vi "pure pursuit.vi"(8 "input cluster":T3={"Drive Forward Input "=0.0, "Drive Twist Input"=0.0, "Drive Output"=0.0, "Drivetwist Output"=0.0, "Left Joystick Buttons"=[FALSE, FALSE, FALSE, FALSE, FALSE, FALSE, FALSE, FALSE, FALSE, FALSE, FALSE, FALSE], "Left Joystick Axis"=[-0.007874015748031496, -0.007874015748031496, -0.0, -1.0], "Right Joystick Axis"=[], "Right Joystick Button"=[], "Arm Encoder"=102.0, "Left Drive Encoder"=2433.0, "Right Drive Encoder"=6910.0, "Gyro Angle "=3.1201171875, "Arm Joystick Output  "=0.0, "Line Follower L, C, R "=[TRUE, TRUE, TRUE], "Line follow?"=FALSE, " Climb Solenoid"=FALSE, "Wrist Encoder Count"=0.0, "Wrist Joystick Output"=0.0, "Ball Encoder Count"=0.0, "Ball Output"=0.0, "Climb Encoder"=0.0, "Climb Motor Output"=0.0, " Hatch Solenoid"=FALSE, "Arm Setpoint "=6.0, "Wrist Setpoint "=0.0, "Arm Joystick Enabled?"=FALSE, "Wrist Joystick Enabled"=FALSE, "Vision String"="", "Left Joystick POVs"=[-1]}, 10 "Vision Data":dbl[](array[numeric]), 11 "Button":bool) -> ()   [LabVIEW 2018]
uses:
  TypeDefs/Teleop Data Cluster.ctl
  path data.ctl
  TypeDefs/typedef_enum_Refnums.ctl
  <vilib>/Rock Robotics/WPI/Utilities/WPI_GetSetVariantRefNum.vi
  <vilib>/Rock Robotics/Network Tables/NT Write Number.vi
  <vilib>/Rock Robotics/WPI/RobotDrive/WPI_RobotDriveArcadeDrive_Standard(NoSaturation).vi
  <vilib>/Rock Robotics/WPI/ThirdParty/Phoenix-LabVIEW/Pigeon IMU/CTRE_PigeonIMU_GetYPR.vi
  <vilib>/ptbypt/NI_PtbyPt.lvlib
panel:
  in  "Extension Weight":dbl=40.0
  in  "Vision Data 2":dbl[](array[numeric])=[100.0, 30.0, 30.0]
  in  "Reverse?":bool
  in  "End Weight":dbl=40.0
  in  "Start Weight":dbl=40.0
  in  "Path Data":T1={"Path"=[], "Target Velocities"=[], "Robot Location"=[0.0, 0.0], "Relative Robot Angle (rad)"=0.0, "Curvature"=0.0, "Lookahead Point"=[0.0, 0.0], "Lookahead Index"=0.0, "Closest Point"=[0.0, 0.0], "Closest Point Index"=0, "Left Velocity"=0.0, "Right Velocity"=0.0, "Left Encoder Vel"=0, "Right Encoder Vel"=0, "Left Encoder Pos"=0, "Right Encoder Pos"=0, "Inital Robot Angle (deg)"=0.0}
  out "error out":errorcluster
  in  "error in":errorcluster
  in  "Diagnostic?":bool=TRUE
  in  "Tuning":T2={"Kv Left"=0.00023, "Kv Right"=0.00023, "Kp Left"=0.0002, "Kp Right"=0.0002}
  out "Loop Time":u32=49
  out "Exp. Curvature":dbl[](graph)=[0.0, 2.1457073059547978e-06, 4.915984271433975e-06, 9.188824286615022e-06, 1.6525472937545946e-05, 3.010957284935173e-05, 5.6788339571684504e-05, 8.289028577213488e-05, 4.477325703165674e-05, 2.456450460867463e-05, 1.378521585638589e-05, 7.731043410757915e-06, 4.074850806979229e-06, 1.5874818402303252e-06, 4.987974022052938e-07, 2.8449815610461093e-06, 6.3492936805341935e-06, 1.2856441230110154e-05, 2.7535758537289207e-05, 3.0160147141967202e-05, 1.4511775279263373e-05, 7.708104280674182e-06, 4.314732936015046e-06, 2.452638698362967e-06, 1.3278260165247803e-06, 5.18742643953799e-07, 0.0]
  out "Curvature":dbl(graph)=-0.0001411444266515344
  out "Target Velocities":cluster{dbl, dbl}(graph)
  in  "Lookahead Distance":dbl=5000.0 format="%#_13g"
  out "Path":T4(graph)=[{"Smooth Path"=[0.0, 183.6988592949273, 380.76323574317996, 607.8995296360172, 889.3325158488149, 1262.8611917273658, 1789.308518427094, 2567.7266854376426, 3771.076875333013, 5232.402820741672, 6849.244028409719, 8558.017396302117, 10318.123190930659, 12101.795305964908, 13887.15873864522, 15652.761438127307, 17372.21087078327, 19007.57686157632, 20499.90780396381, 21754.493387203354, 23022.702335030026, 24295.5868812136, 25565.368128084057, 26823.491402011234, 28058.487557976674, 29253.105583025565, 30379.999999999993], "Smooth Path"=[0.0, 2562.5448292081915, 5114.539619045078, 7642.796141488607, 10128.191737636604, 12540.888817075378, 14832.875496937382, 16925.961760858292, 18910.53913716453, 20828.576963041232, 22705.412156107523, 24556.078957478312, 26389.070280301727, 28208.460788155666, 30014.92415836178, 31805.902606457305, 33574.96665674355, 35310.20911679595, 36991.26656448049, 38584.22946121987, 40426.874048932084, 42415.21298923889, 44481.68243571063, 46578.25117050202, 48664.41284268002, 50697.05928458697, 52619.7035339425]}, {"Smooth Path"=[24052.273982374318, 27574.516343499825], "Smooth Path"=[40888.03333583952, 45745.37919026383]}, {"Smooth Path"=[30379.999999999993, 24052.273982374318], "Smooth Path"=[52619.7035339425, 40888.03333583952]}]
  in  "Config":T5={"Path"={"Spacing"=2608.0, "Smooth Weight"=0.8, "Tolerance"=0.01}, "Kinematics"={"Max Vel"=1250.0, "Max Accel"=200.0, "Curvature Const"=0.1}}
  in  "Waypoints":dbl[][](array[numeric])=[[0.0, 0.0], [2.0, 30000.0], [20000.0, 60000.0]]
  in  "Track Width":dbl=14000.0 format="%#_13g"
  out "Right Output":dbl=0.02
  out "Left Output":dbl=0.0058000000000000005
  out "Left Velocity":T6(graph)={"Quadrature Velocity"=-29, "Left Velocity"=0.0}
  out "Right Velocity":T7(graph)={"Quadrature Velocity"=-100, "Right Velocity"=0.0}
  out "Robot Angle":dbl=35.947265625
  out "Curvature":dbl=-0.0001411444266515344
  out "Robot Location":dbl[](array[numeric])=[24052.273982374318, 40888.03333583952]
  out "Right Velocity":dbl
  out "Left Velocity":dbl
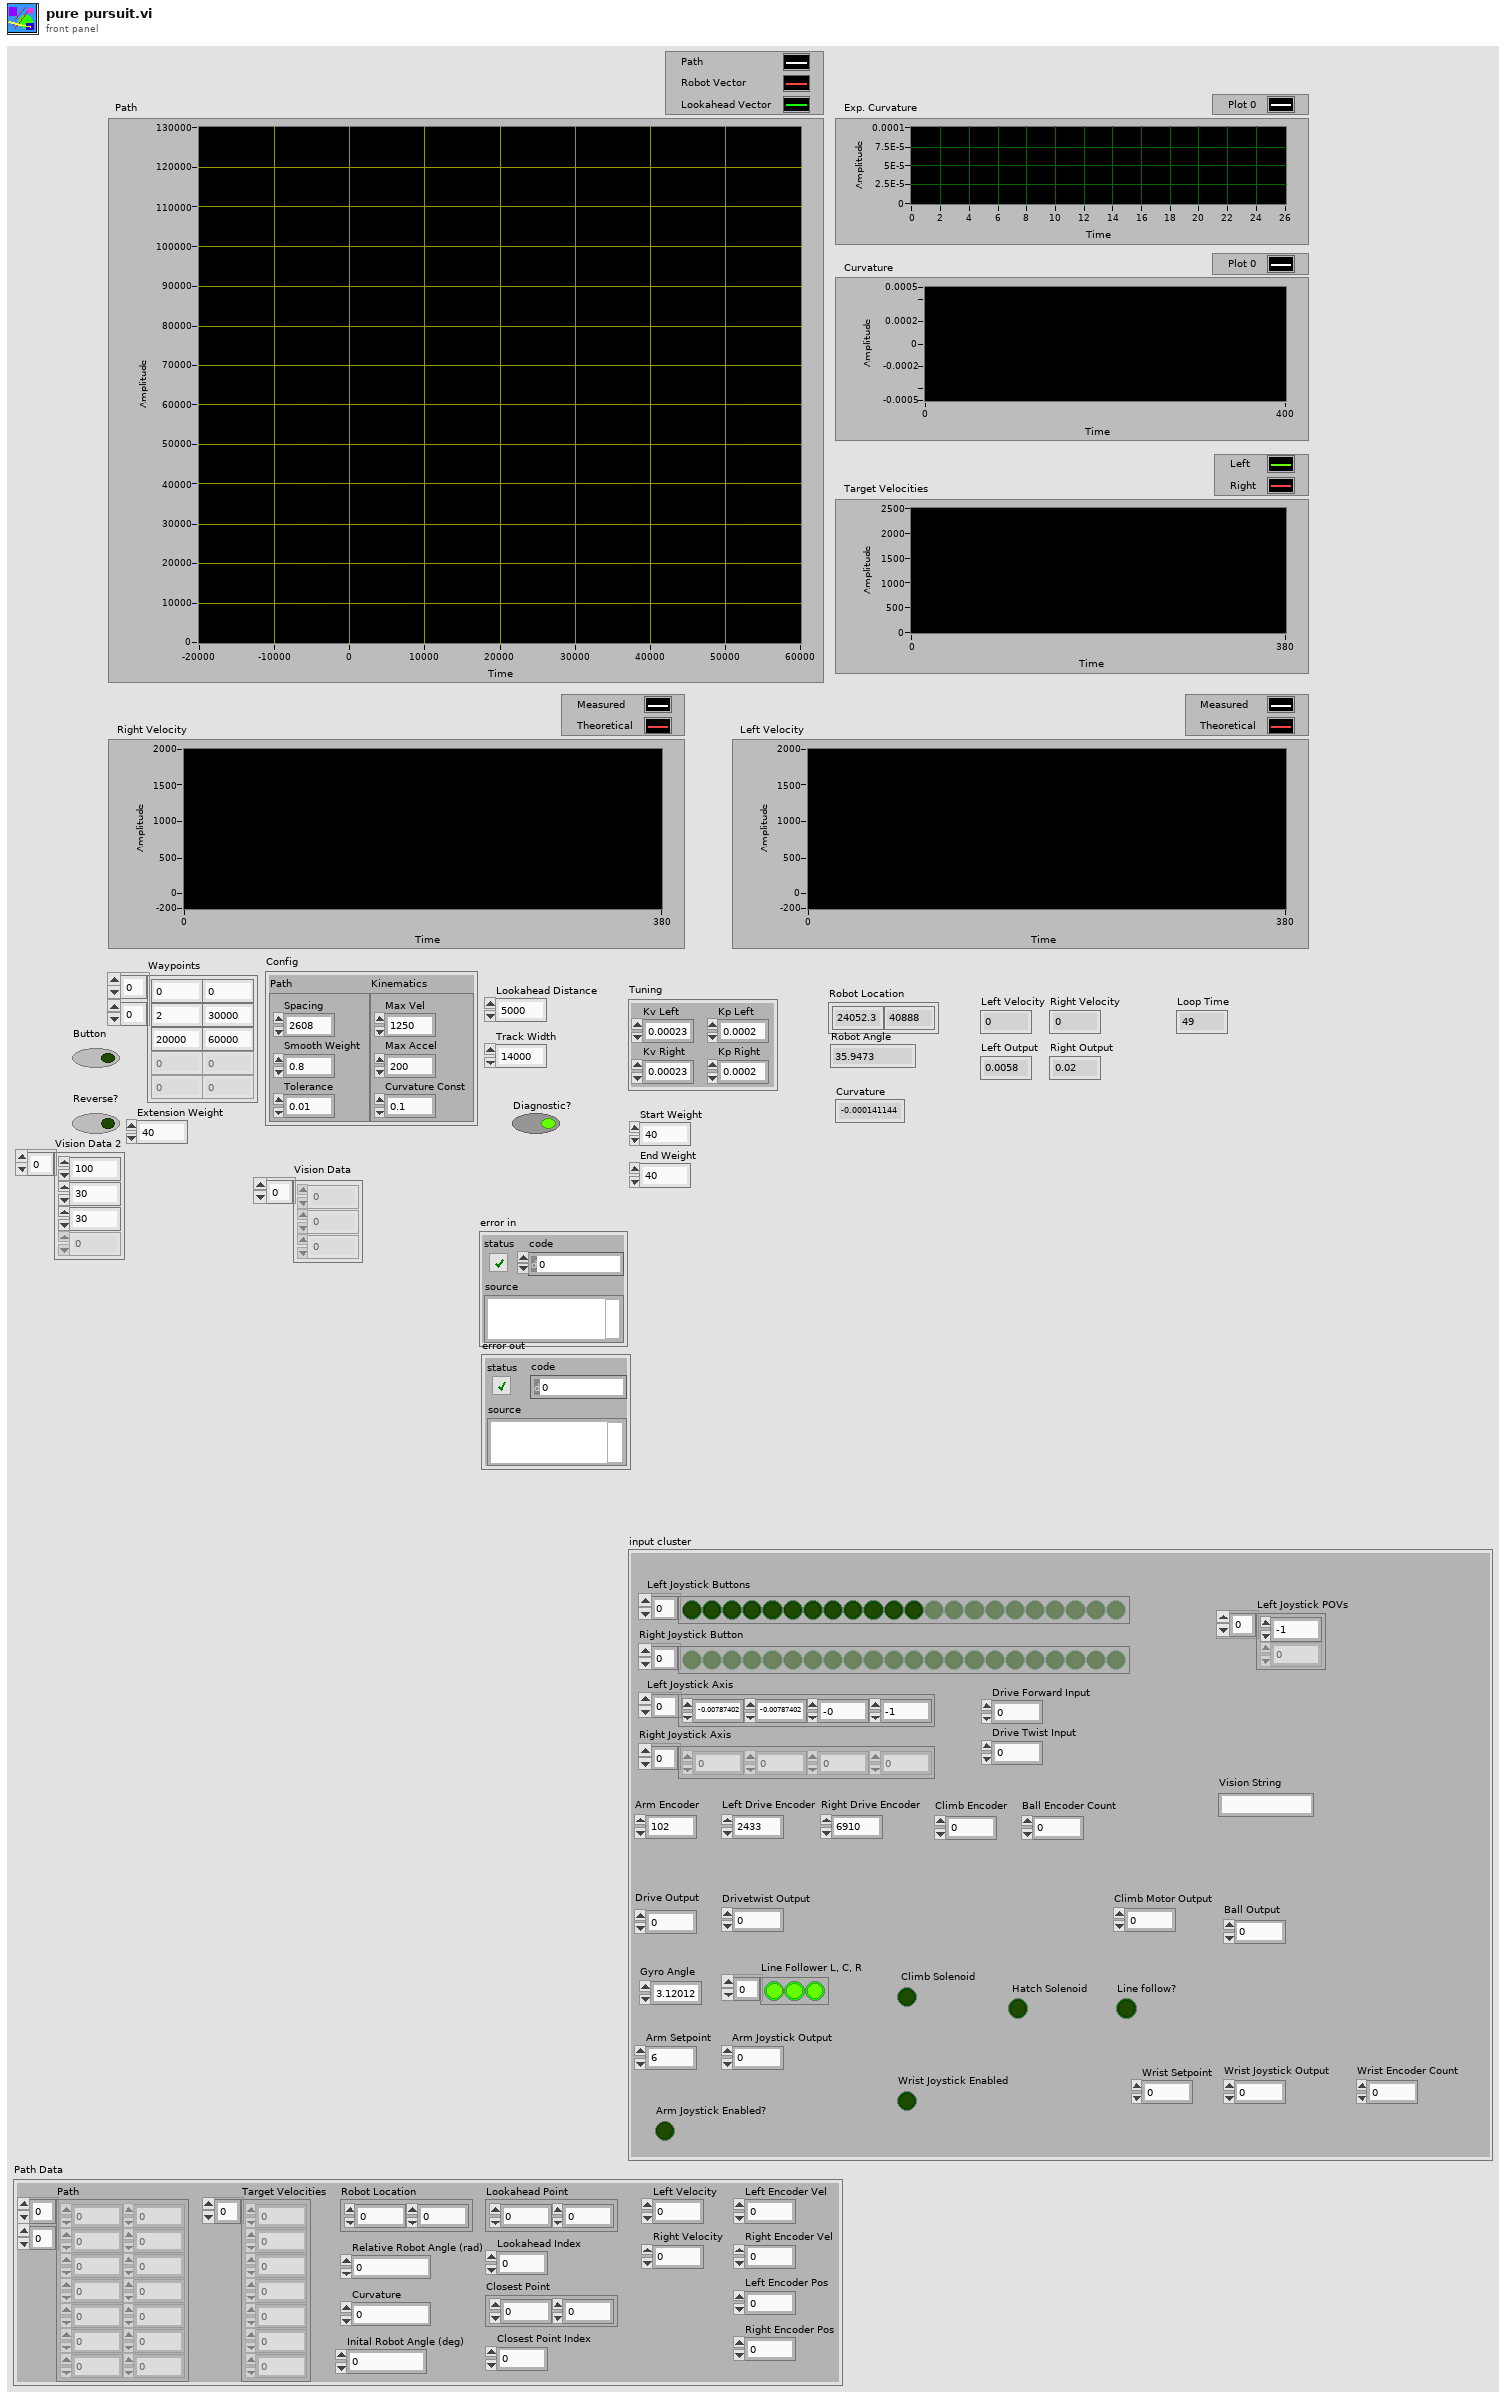
[diagram p1: front panel]
types:
  T1 = typedef "path data.ctl" = cluster{"Path":dbl[][], "Target Velocities":dbl[], "Robot Location":dbl[], "Relative Robot Angle (rad)":dbl, "Curvature":dbl, "Lookahead Point":dbl[], "Lookahead Index":dbl, "Closest Point":dbl[], "Closest Point Index":i32, "Left Velocity":dbl, "Right Velocity":dbl, "Left Encoder Vel":i32, "Right Encoder Vel":i32, "Left Encoder Pos":i32, "Right Encoder Pos":i32, "Inital Robot Angle (deg)":dbl}
  T2 = cluster{"Kv Left":dbl, "Kv Right":dbl, "Kp Left":dbl, "Kp Right":dbl}
  T3 = typedef "Teleop Data Cluster.ctl" = cluster{"Drive Forward Input ":dbl, "Drive Twist Input":dbl, "Drive Output":dbl, "Drivetwist Output":dbl, "Left Joystick Buttons":bool[], "Left Joystick Axis":dbl[], "Right Joystick Axis":dbl[], "Right Joystick Button":bool[], "Arm Encoder":dbl, "Left Drive Encoder":dbl, "Right Drive Encoder":dbl, "Gyro Angle ":dbl, "Arm Joystick Output  ":dbl, "Line Follower L, C, R ":bool[], "Line follow?":bool, " Climb Solenoid":bool, "Wrist Encoder Count":dbl, "Wrist Joystick Output":dbl, "Ball Encoder Count":dbl, "Ball Output":dbl, "Climb Encoder":dbl, "Climb Motor Output":dbl, " Hatch Solenoid":bool, "Arm Setpoint ":dbl, "Wrist Setpoint ":dbl, "Arm Joystick Enabled?":bool, "Wrist Joystick Enabled":bool, "Vision String":string, "Left Joystick POVs":i16[]}
  T4 = cluster{"Smooth Path":dbl[], "Smooth Path":dbl[]}[]
  T5 = cluster{"Path":cluster{"Spacing":dbl, "Smooth Weight":dbl, "Tolerance":dbl}, "Kinematics":cluster{"Max Vel":dbl, "Max Accel":dbl, "Curvature Const":dbl}}
  T6 = cluster{"Quadrature Velocity":i32, "Left Velocity":dbl}
  T7 = cluster{"Quadrature Velocity":i32, "Right Velocity":dbl}
  T8 = typedef "typedef_enum_Refnums.ctl" = enum16{"Ball_Encoder", "Ball_Motor", "Camera", "Linefollow_3", "Linefollow_2", "Linefollow_1", "Gyro", "Hatch_Solenoid", "Climb_Back_Solenoid", "Arm_Encoder", "Arm_Motor", "Lift_Encoder", "Drive", "Drive_Motor_R", "Drive_Motor_L", "Drive_Encoder_R", "Drive_Encoder_L", "Joy_R", "Joy_L", "Wrist_Motor", "Wrist_Encoder", "Climb Upper Limit", "Climb Lower Limit ", "Climb_Front_Motor"}
  T9 = typedef "WPI_RobotDriveDevRef.ctl" = cluster{"DevStatus":errorcluster, "Motors[]":T10[], "Square Inputs":bool, "Max Output":dbl}
  T10 = typedef "WPI_MotorControlDeviceRef.ctl" = cluster{"DeviceStatus":errorcluster, "Type":T11, "PWM":cluster{"PWM Channel":T12, "DeadBand":T13}, "CAN":cluster{"Device Number":u8, "SetOutput VI Ref":variant, "GetOutput VI Ref":variant, "Enable VI Ref":variant, "Disable VI Ref":variant, "Data":variant}, "Invert":bool, "DIO PWM":cluster{"PWM \"Enable\" Channel":T12, "DIOChannel":T14, "PWM Rate":dbl}}
  T11 = typedef "WPI_MotorControlType.ctl" = enum16{"PWM", "CAN", "DIO PWM"}
  T12 = typedef "FPGA_DIOPWMChannel.ctl" = enum8{"PWM 0", "PWM 1", "PWM 2", "PWM 3", "PWM 4", "PWM 5", "PWM 6", "PWM 7", "PWM 8", "PWM 9", "PWM MXP 0", "PWM MXP 1", "PWM MXP 2", "PWM MXP 3", "PWM MXP 4", "PWM MXP 5", "PWM MXP 6", "PWM MXP 7", "PWM MXP 8", "PWM MXP 9", "Invalid"}
  T13 = typedef "WPI_PWMDeadband.ctl" = cluster{"Name":string, "maxPositivePwm":i32, "minPositivePwm":i32, "centerPwm":i32, "maxNegativePwm":i32, "minNegativePwm":i32, "angularRange":u16}
  T14 = typedef "FPGA_DIOChannel.ctl" = enum8{"DIO 0", "DIO 1", "DIO 2", "DIO 3", "DIO 4", "DIO 5", "DIO 6", "DIO 7", "DIO 8", "DIO 9", "DIO MXP 0", "DIO MXP 1", "DIO MXP 2", "DIO MXP 3", "DIO MXP 4", "DIO MXP 5", "DIO MXP 6", "DIO MXP 7", "DIO MXP 8", "DIO MXP 9", "DIO MXP 10", "DIO MXP 11", "DIO MXP 12", "DIO MXP 13", "DIO MXP 14", "DIO MXP 15", "SPI Port CS1", "SPI Port CS2", "SPI Port CS3", "SPI Port MISO", "SPI Port MOSI", "Invalid"}
  T15 = typedef "CTRE_PigeonIMU_DeviceRef.ctl" = cluster{"DeviceStatus":errorcluster, "Device Number":u8, "Type":T16, "Device ID":u32, "Handle":u64, "UsageFrame":u32, "Library Path":path}
  T16 = typedef "CTRE_PigeonIMU_ConnectionType.ctl" = u32
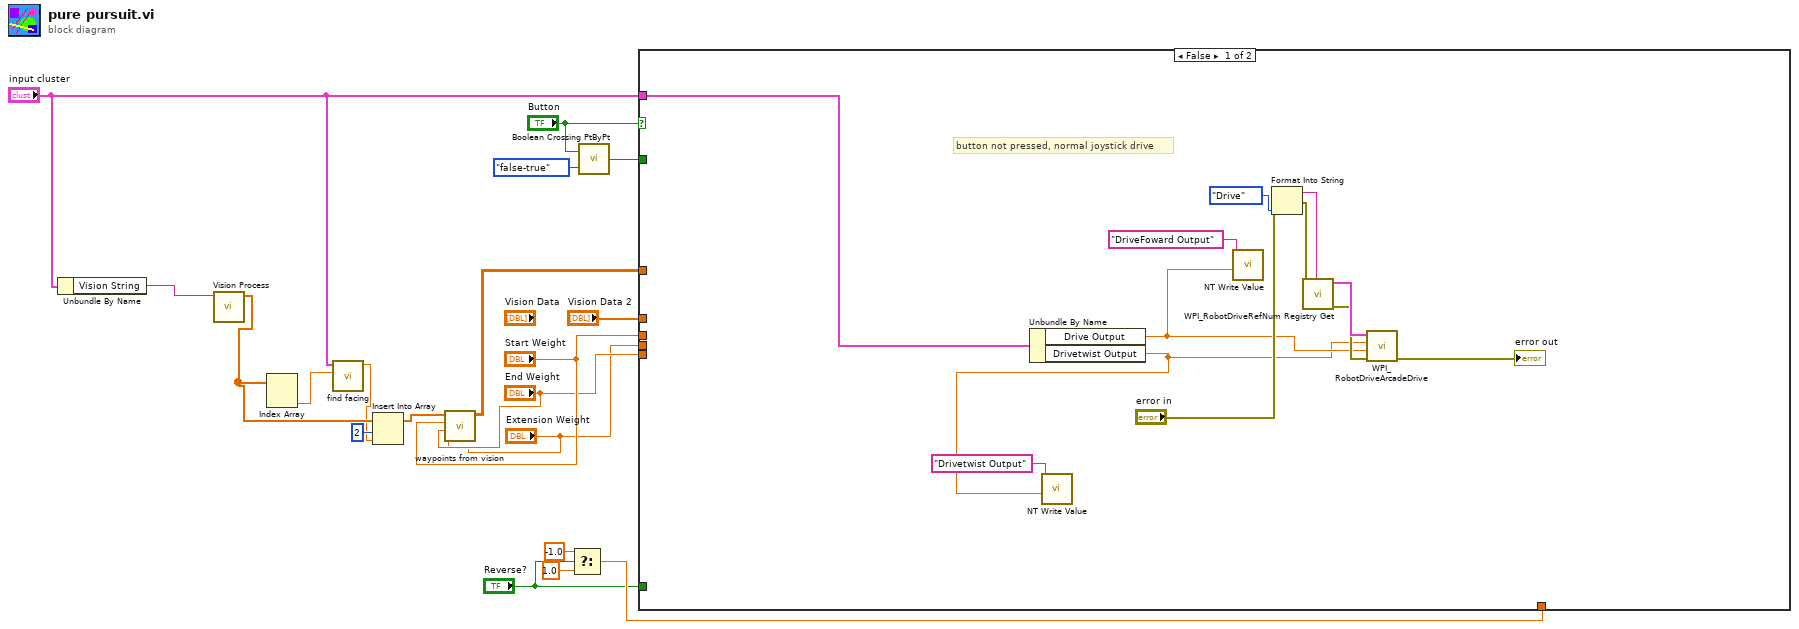
[diagram p0: block diagram]
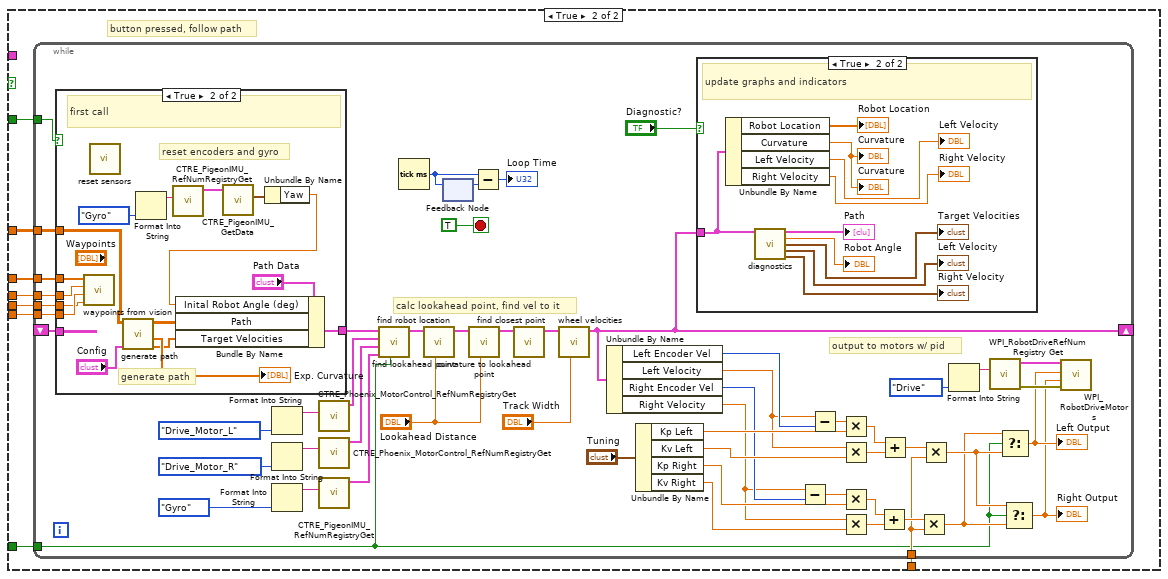
[diagram p2: hidden frame]
diagram:
  n1 = Unbundle By Name("input cluster") -> ("Vision String"=w8:string)
  n2 = call "Vision Process.vi"("Vision String"=w8) -> ("Default Values"=w7:dbl[])  [unwired: 10 in]
  n3 = Index Array(array=w7) -> (element #2=w11:dbl)  [unwired: 2 in, 1 out]
  n4 = call "find facing.vi"("Robot Angle"=w11, "TeleOp Data Cluster"="input cluster") -> ("Facing"=w1:dbl)  [unwired: 9 in]
  n5 = Insert Into Array(array=w7, index=2, new element=w1) -> (w9:dbl[])
  n6 = call "waypoints from vision.vi"("Extension Weight"="Extension Weight", "End Weight"="End Weight", "Start Weight"="Start Weight", "Vision Data"=w9) -> ("Waypoints"=w6:dbl[][])  [unwired: 7 in]
  n7 = Select(t=-1.0, s="Reverse?", f=1.0) -> (s? t:f=w14:dbl)
  n8 = call <vilib>:"Boolean Crossing PtByPt.vi"("direction"=enum16{"either", "false-true", "true-false"}."false-true", "input"="Button") -> ("crossing"=w17:bool)  [unwired: 1 in]
  n9 = case shown="False" "Button" {
    tunnel: w17 -> [_ w39]
    tunnel: "Vision Data 2" -> [_ w38]
    tunnel: w14 -> [_ w37]
    tunnel: "Reverse?" -> [_ w36]
    tunnel: "End Weight" -> [_ w35]
    tunnel: "Start Weight" -> [_ w34]
    tunnel: "Extension Weight" -> [_ w33]
    tunnel: "input cluster" -> [w22 _]
    tunnel: w6 -> [_ w32]
    frame False {
      # "button not pressed, normal joystick drive"
      n10 = Unbundle By Name(w22) -> ("Drive Output"=w24:dbl, "Drivetwist Output"=w20:dbl)
      n11 = call-poly <vilib>:"NT Write Value.vi"("Numeric"=w20, "Name"="Drivetwist Output") -> ()  [unwired: 9 in, 1 out]
      n12 = call-poly <vilib>:"NT Write Value.vi"("Numeric"=w24, "Name"="DriveFoward Output") -> ()  [unwired: 9 in, 1 out]
      n13 = Format Into String(error in="error in", typedef_enum_Refnums."Drive" ("RefNums")) -> (resulting string=w30:string, error out=w27:errorcluster)  [unwired: 2 in]
      n14 = call <vilib>:"WPI_RobotDriveRefNum Registry Get.vi"("error in (no error)"=w27, "refnum name"=w30) -> ("error out"=w26:errorcluster, "RobotDriveDevRef"=w31:T9)  [unwired: 8 in]
      n15 = call-poly <vilib>:"WPI_RobotDriveArcadeDrive.vi"("error in (no error)"=w26, "Y axis value"=w24, "X axis value"=w20, "RobotDriveDevRef"=w31) -> ("error out"=→"error out":errorcluster)  [unwired: 5 in, 2 out]
    }
    frame True {
      # "button pressed, follow path"
      n16 = while {
        tunnel: w39 -> [w59]
        shift-right: [w61] -> _
        shift-left: _ -> [w70]
        tunnel: w38 -> [w50]
        tunnel: w37 -> [w49]
        tunnel: w36 -> [w44]
        tunnel: w35 -> [w43]
        tunnel: w34 -> [w42]
        tunnel: w33 -> [w41]
        tunnel: w32 -> [w40]
        stop <- TRUE stop-if-true
        # "calc lookahead point, find vel to it"
        # "output to motors w/ pid"
        n17 = case shown="True" w59 {
          tunnel: [w106 w118] -> w60
          tunnel: w70 -> [w106 _]
          tunnel: w50 -> [_ w117]
          tunnel: w43 -> [_ w116]
          tunnel: w42 -> [_ w115]
          tunnel: w41 -> [_ w108]
          tunnel: w40 -> [_ w107]
          frame False {
          }
          frame True {
            # "generate path"
            # "reset encoders and gyro"
            # "first call"
            n18 = call "waypoints from vision.vi"("Extension Weight"=w108, "End Weight"=w116, "Start Weight"=w115, "Vision Data"=w117) -> ()  [unwired: 7 in, 1 out]
            n19 = call "reset sensors.vi"() -> ()  [unwired: 12 in]
            n20 = call "generate path.vi"("Config"="Config", "Waypoints"=w107) -> ("Target Velocities"=w112:dbl[], "Curvatures"=→"Exp. Curvature":dbl[], "Smooth Path"=w119:dbl[][])  [unwired: 4 in, 3 out]
            n21 = Format Into String(typedef_enum_Refnums."Gyro" ("RefNums")) -> (resulting string=w113:string)  [unwired: 3 in, 1 out]
            n22 = call <vilib>:"CTRE_PigeonIMU_RefNumRegistryGet.vi"("refnum name"=w113) -> ("PigeonIMUDevRef"=w111:T15)  [unwired: 9 in, 1 out]
            n23 = call-poly <vilib>:"CTRE_PigeonIMU_GetData.vi"("PigeonIMUDevRef"=w111) -> ("Yaw Pitch Roll"=w110:cluster{"Yaw":dbl, "Pitch":dbl, "Roll":dbl})  [unwired: 8 in, 2 out]
            n24 = Unbundle By Name(w110) -> ("Yaw"=w109:dbl)
            n25 = Bundle By Name(cluster="Path Data", "Inital Robot Angle (deg)"=w109, "Path"=w119, "Target Velocities"=w112) -> (w118:T1)
          }
        }
        n26 = Format Into String(typedef_enum_Refnums."Drive_Motor_L" ("RefNums")) -> (resulting string=w55:string)  [unwired: 3 in, 1 out]
        n27 = Format Into String(typedef_enum_Refnums."Drive_Motor_R" ("RefNums")) -> (resulting string=w54:string)  [unwired: 3 in, 1 out]
        n28 = Format Into String(typedef_enum_Refnums."Gyro" ("RefNums")) -> (resulting string=w53:string)  [unwired: 3 in, 1 out]
        n29 = call <vilib>:"CTRE_Phoenix_MotorControl_RefNumRegistryGet.vi"("refnum name"=w55) -> ("PhoenixMotorControlDevRef"=w66:T10)  [unwired: 9 in, 1 out]
        n30 = call <vilib>:"CTRE_Phoenix_MotorControl_RefNumRegistryGet.vi"("refnum name"=w54) -> ("PhoenixMotorControlDevRef"=w67:T10)  [unwired: 9 in, 1 out]
        n31 = call <vilib>:"CTRE_PigeonIMU_RefNumRegistryGet.vi"("refnum name"=w53) -> ("PigeonIMUDevRef"=w68:T15)  [unwired: 9 in, 1 out]
        n32 = call "find robot location.vi"("Reverse?"=w44, "Pigeon Reference"=w68, "Right Encoder Reference"=w67, "Left Encoder Reference"=w66, "Path Data"=w60) -> ("Path Data"=w69:T1)  [unwired: 6 in]
        n33 = Tick Count (ms)() -> (millisecond timer value=w87:u32)
        n34 = call "find lookahead point.vi"("Lookahead Distance"="Lookahead Distance", "Path Data"=w69) -> ("Path Data"=w73:T1)  [unwired: 9 in]
        n35 = feedback-in #1(w87) -> ()
        n36 = feedback #1() -> (w86:u32)  [unwired: 1 in]
        n37 = call "curvature to lookahead point.vi"("Lookahead Distance"="Lookahead Distance", "Path Data"=w73) -> ("Path Data"=w72:T1)  [unwired: 9 in]
        n38 = Subtract(x=w87, y=w86) -> (x-y=→"Loop Time":u32)
        n39 = call "find closest point.vi"("Path Data"=w72) -> ("Path Data"=w71:T1)  [unwired: 10 in]
        n40 = call "wheel velocities.vi"("Track Width"="Track Width", "Path Data"=w71) -> ("Path Data"=w61:T1)  [unwired: 9 in]
        n41 = Unbundle By Name(w61) -> ("Left Encoder Vel"=w65:i32, "Left Velocity"=w64:dbl, "Right Encoder Vel"=w63:i32, "Right Velocity"=w62:dbl)
        n42 = Unbundle By Name("Tuning") -> ("Kp Left"=w81:dbl, "Kv Left"=w80:dbl, "Kp Right"=w79:dbl, "Kv Right"=w78:dbl)
        n43 = case shown="True" "Diagnostic?" {
          tunnel: w61 -> [_ w96]
          frame False {
          }
          frame True {
            # "update graphs and indicators"
            n44 = Unbundle By Name(w96) -> ("Robot Location"=→"Robot Location":dbl[], "Curvature"=→"Curvature" →"Curvature":dbl, "Left Velocity"=→"Left Velocity":dbl, "Right Velocity"=→"Right Velocity":dbl)
            n45 = call "diagnostics.vi"("Path Data"=w96) -> ("Path"=→"Path":T4, "Robot Angle (deg)"=→"Robot Angle":dbl, "Target Velocities"=→"Target Velocities":cluster{dbl, dbl}, "Left Velocity"=→"Left Velocity":T6, "Right Velocity"=→"Right Velocity":T7)  [unwired: 10 in]
          }
        }
        n46 = Subtract(x=w62, y=w63) -> (x-y=w89:dbl)
        n47 = Subtract(x=w64, y=w65) -> (x-y=w91:dbl)
        n48 = Multiply(x=w91, y=w81) -> (x*y=w90:dbl)
        n49 = Multiply(x=w64, y=w80) -> (x*y=w93:dbl)
        n50 = Multiply(x=w89, y=w79) -> (x*y=w88:dbl)
        n51 = Multiply(x=w62, y=w78) -> (x*y=w92:dbl)
        n52 = Add(x=w88, y=w92) -> (x+y=w84:dbl)
        n53 = Add(x=w90, y=w93) -> (x+y=w83:dbl)
        n54 = Multiply(x=w84, y=w49) -> (x*y=w45:dbl)
        n55 = Multiply(x=w83, y=w49) -> (x*y=w46:dbl)
        n56 = Format Into String(typedef_enum_Refnums."Drive" ("RefNums")) -> (resulting string=w51:string)  [unwired: 3 in, 1 out]
        n57 = call <vilib>:"WPI_RobotDriveRefNum Registry Get.vi"("refnum name"=w51) -> ("error out"=w75:errorcluster, "RobotDriveDevRef"=w74:T9)  [unwired: 9 in]
        n58 = Select(t=w45, s=w44, f=w46) -> (s? t:f=w48:dbl)
        "Left Output" <- w48
        n59 = Select(t=w46, s=w44, f=w45) -> (s? t:f=w47:dbl)
        "Right Output" <- w47
        n60 = call <vilib>:"WPI_RobotDriveMotors.vi"("error in (no error)"=w75, "RightSpeed"=w47, "LeftSpeed"=w48, "RobotDriveDevRef"=w74) -> ()  [unwired: 5 in, 3 out]
      }
    }
  }
